vi "Get Route Group Specifications.vi"(8 "error in (no error)":errorcluster, 11 "Virtual Device Name":string="PPack_B_Test") -> (0 "error out":errorcluster, 1 "IVI Names":string[][](array[string]), 3 "Specifications":string[][](array[string]))   [LabVIEW 2019]
uses:
  <vilib>/SwitchExecutive/niseCfg.llb/niseCfg Get Virtual Device.vi
  <vilib>/SwitchExecutive/niseCfg.llb/niseVirtualDevice Get Route Groups.vi
panel:
  out "Route Name":string[](array[string])
  out "Count":i32
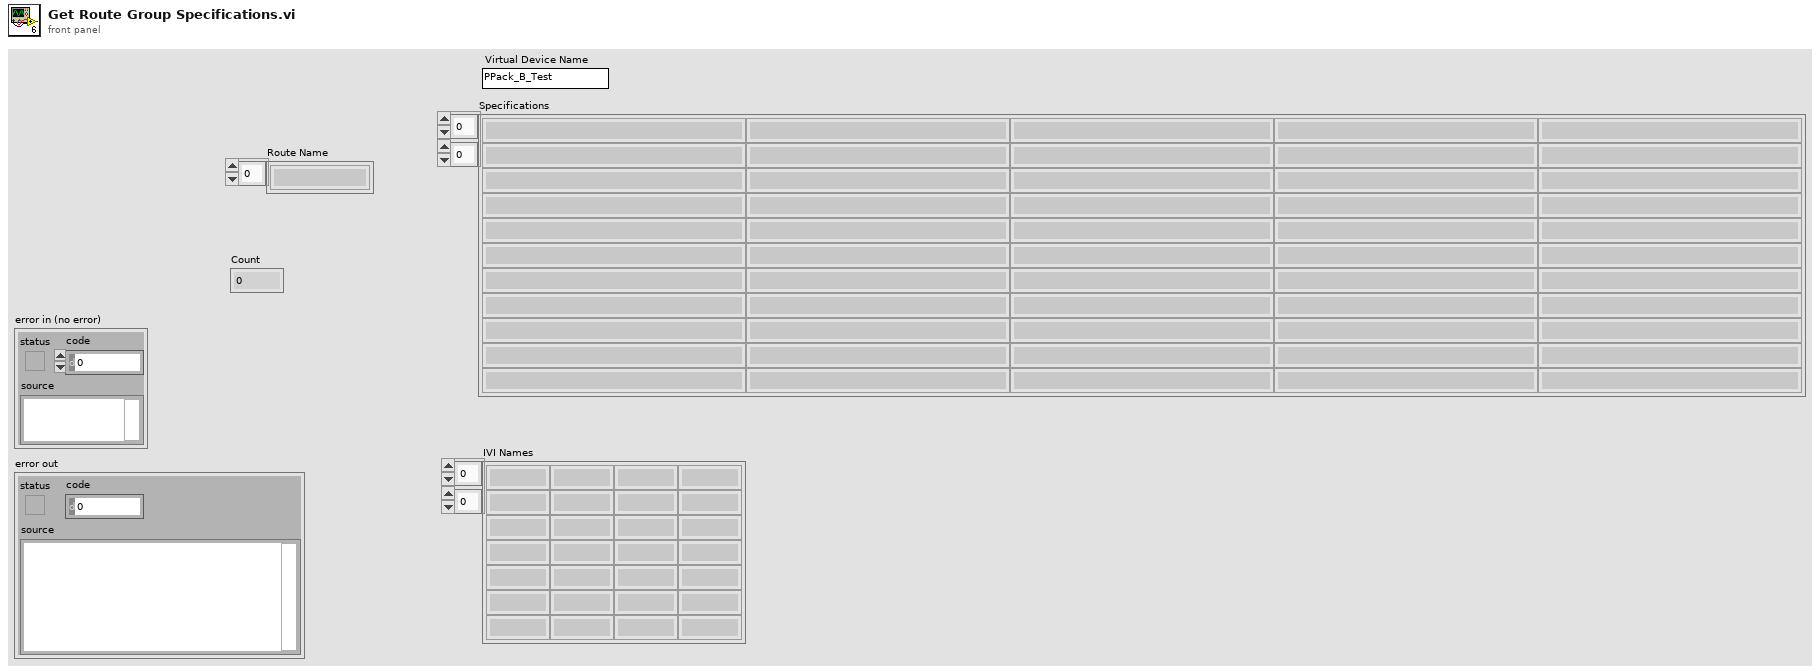
[diagram p1: front panel]
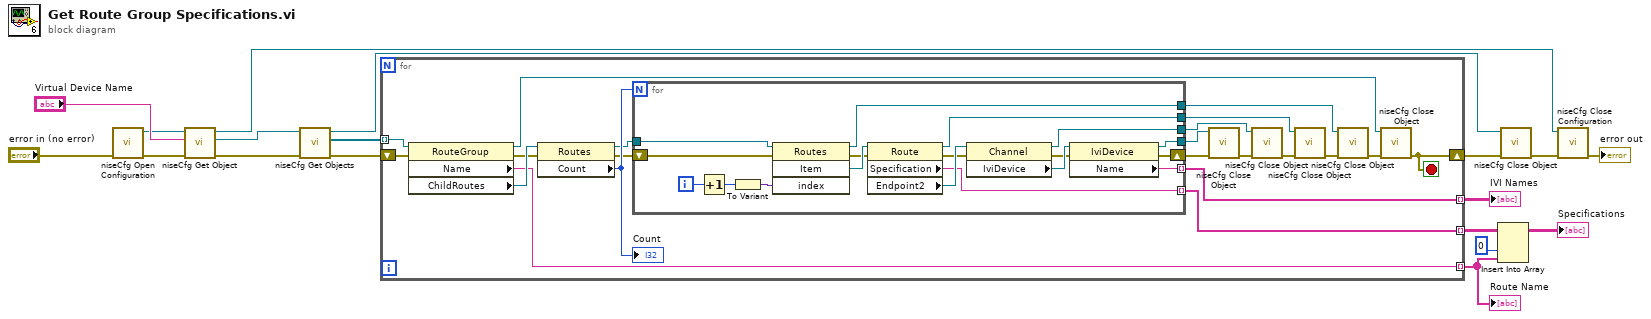
[diagram p0: block diagram]
diagram:
  n1 = call <vilib>:"niseCfg Open Configuration.vi"("error in (no error)"="error in (no error)") -> ("error out"=w18:errorcluster, "niseCfg"=w15:refnum<k7>)  [unwired: 9 in]
  n2 = call-poly <vilib>:"niseCfg Get Object.vi"("error in (no error)"=w18, "Virtual Device Name"="Virtual Device Name", "niseCfg"=w15) -> ("error out"=w6:errorcluster, "Virtual Device"=w7:refnum<k7>, "niseCfg out"=w16:refnum<k7>)  [unwired: 6 in]
  n3 = call-poly <vilib>:"niseCfg Get Objects.vi"("error in (no error)"=w6, "Virtual Device"=w7) -> ("error out"=w13:errorcluster, "Route Groups"=w14:refnum<k7>[], "Virtual Device out"=w12:refnum<k7>)  [unwired: 7 in]
  n4 = for {
    tunnel: w14 -> [w35] mode=indexing
    shift-right: [w20] -> w10
    shift-left: w13 -> [w34]
    tunnel: [w22] -> w5 mode=indexing
    tunnel: [w21] -> w4 mode=indexing
    tunnel: [w19] -> w2 mode=indexing
    stop <- w20 stop-if-true
    n5 = property class="RouteGroup"(reference=w35, error in=w34) -> (reference out=w26:refnum<k7>, error out=w33:errorcluster, "Name"=w19:string, "ChildRoutes"=w37:refnum<k7>)
    n6 = property class="Routes"(reference=w37, error in=w33) -> (reference out=w27:refnum<k7>, error out=w32:errorcluster, "Count"=w36:i32)
    "Count" <- w36
    n7 = for {
      N: w36 -> [_]
      tunnel: w27 -> [w57]
      tunnel: [w49] -> w21 mode=indexing
      tunnel: [w48] -> w22 mode=indexing
      shift-right: [w47] -> w25
      shift-left: w32 -> [w54]
      tunnel: [w44] -> w31
      tunnel: [w43] -> w30
      tunnel: [w42] -> w29
      tunnel: [w41] -> w28
      i -> [w46]
      n8 = Increment(x=w46) -> (x+1=w40:i32)
      n9 = To Variant(anything=w40) -> (Variant=w45:variant)
      n10 = invoke class="Routes" method="Item"(reference=w57, error in=w54, "index"=w45) -> (reference out=w41:refnum<k7>, error out=w55:errorcluster, "Item"=w56:refnum<k7>)  [unwired: 1 in, 1 out]
      n11 = property class="Route"(reference=w56, error in=w55) -> (reference out=w42:refnum<k7>, error out=w51:errorcluster, "Specification"=w49:string, "Endpoint2"=w53:refnum<k7>)
      n12 = property class="Channel"(reference=w53, error in=w51) -> (reference out=w43:refnum<k7>, error out=w50:errorcluster, "IviDevice"=w52:refnum<k7>)
      n13 = property class="IviDevice"(reference=w52, error in=w50) -> (reference out=w44:refnum<k7>, error out=w47:errorcluster, "Name"=w48:string)
    }
    n14 = call <vilib>:"niseCfg Close Object.vi"("error in (no error)"=w25, "Reference"=w31) -> ("error out"=w24:errorcluster)  [unwired: 9 in]
    n15 = call <vilib>:"niseCfg Close Object.vi"("error in (no error)"=w24, "Reference"=w30) -> ("error out"=w23:errorcluster)  [unwired: 9 in]
    n16 = call <vilib>:"niseCfg Close Object.vi"("error in (no error)"=w23, "Reference"=w29) -> ("error out"=w39:errorcluster)  [unwired: 9 in]
    n17 = call <vilib>:"niseCfg Close Object.vi"("error in (no error)"=w39, "Reference"=w28) -> ("error out"=w38:errorcluster)  [unwired: 9 in]
    n18 = call <vilib>:"niseCfg Close Object.vi"("error in (no error)"=w38, "Reference"=w26) -> ("error out"=w20:errorcluster)  [unwired: 9 in]
  }
  "IVI Names" <- w5
  "Route Name" <- w2
  n19 = Insert Into Array(array=w4, index (col)=0 ("disabled index (col)"), new element=w2) -> (→"Specifications":string[][])  [unwired: 1 in]
  n20 = call <vilib>:"niseCfg Close Object.vi"("error in (no error)"=w10, "Reference"=w12) -> ("error out"=w11:errorcluster)  [unwired: 9 in]
  n21 = call <vilib>:"niseCfg Close Configuration.vi"("error in (no error)"=w11, "niseCfg"=w16) -> ("error out"=→"error out":errorcluster)  [unwired: 9 in]
